vi "试验判定 - 副本.vi"(7 "Result":refnum<vi>, 10 "判定参数":T1, 11 "XY曲线":cluster{"X":dbl[], "Y":dbl[]}[](array[cluster])) -> (2 "判定项长度":i32, 3 "OK？":bool)   [LabVIEW 2020]
uses:
  Global_Variable/A131258.vi
  <userlib>/_MGI/1D Array/MGI Average/MGI Average (DBL[]).vi
panel:
  out "逆向平均值":dbl
  out "正向平均值":dbl
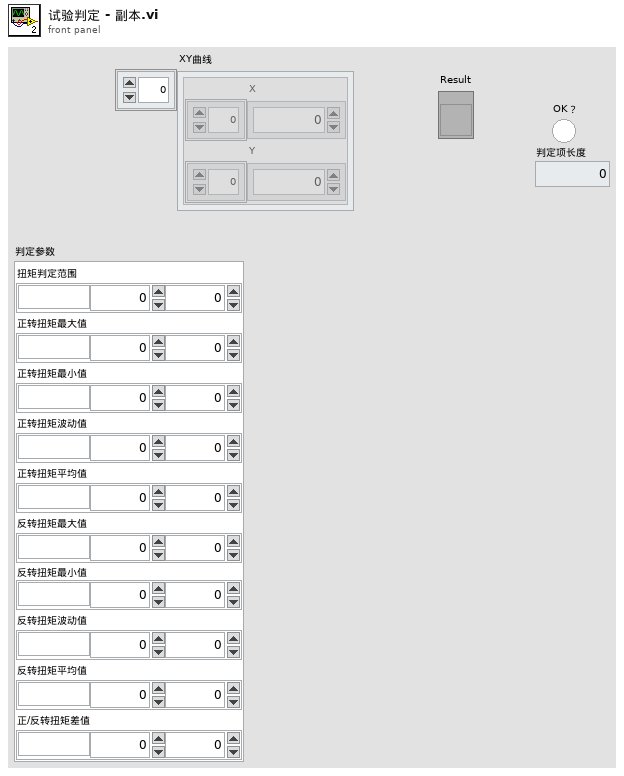
[diagram p1: front panel]
types:
  T1 = cluster{"扭矩判定范围":cluster{"单位":string, "下限":dbl, "上限":dbl}, "正转扭矩最大值":cluster{"单位":string, "下限":dbl, "上限":dbl}, "正转扭矩最小值":cluster{"单位":string, "下限":dbl, "上限":dbl}, "正转扭矩波动值":cluster{"单位":string, "下限":dbl, "上限":dbl}, "正转扭矩平均值":cluster{"单位":string, "下限":dbl, "上限":dbl}, "反转扭矩最大值":cluster{"单位":string, "下限":dbl, "上限":dbl}, "反转扭矩最小值":cluster{"单位":string, "下限":dbl, "上限":dbl}, "反转扭矩波动值":cluster{"单位":string, "下限":dbl, "上限":dbl}, "反转扭矩平均值":cluster{"单位":string, "下限":dbl, "上限":dbl}, "正/反转扭矩差值":cluster{"单位":string, "下限":dbl, "上限":dbl}}
  T2 = cluster{"左平均扭矩":cluster{"正转":dbl, "反转":dbl}, "左矩波动":cluster{"正转":dbl, "反转":dbl}, "左空载":cluster{"正转":dbl, "反转":dbl}, "右平均扭矩":cluster{"正转":dbl, "反转":dbl}, "右扭矩波动":cluster{"正转":dbl, "反转":dbl}, "右空载":cluster{"正转":dbl, "反转":dbl}, "扭矩对称":cluster{"左":dbl, "右":dbl}, "左零点漂移":cluster{"正":dbl, "反":dbl}, "右零点漂移":cluster{"正":dbl, "反":dbl}}
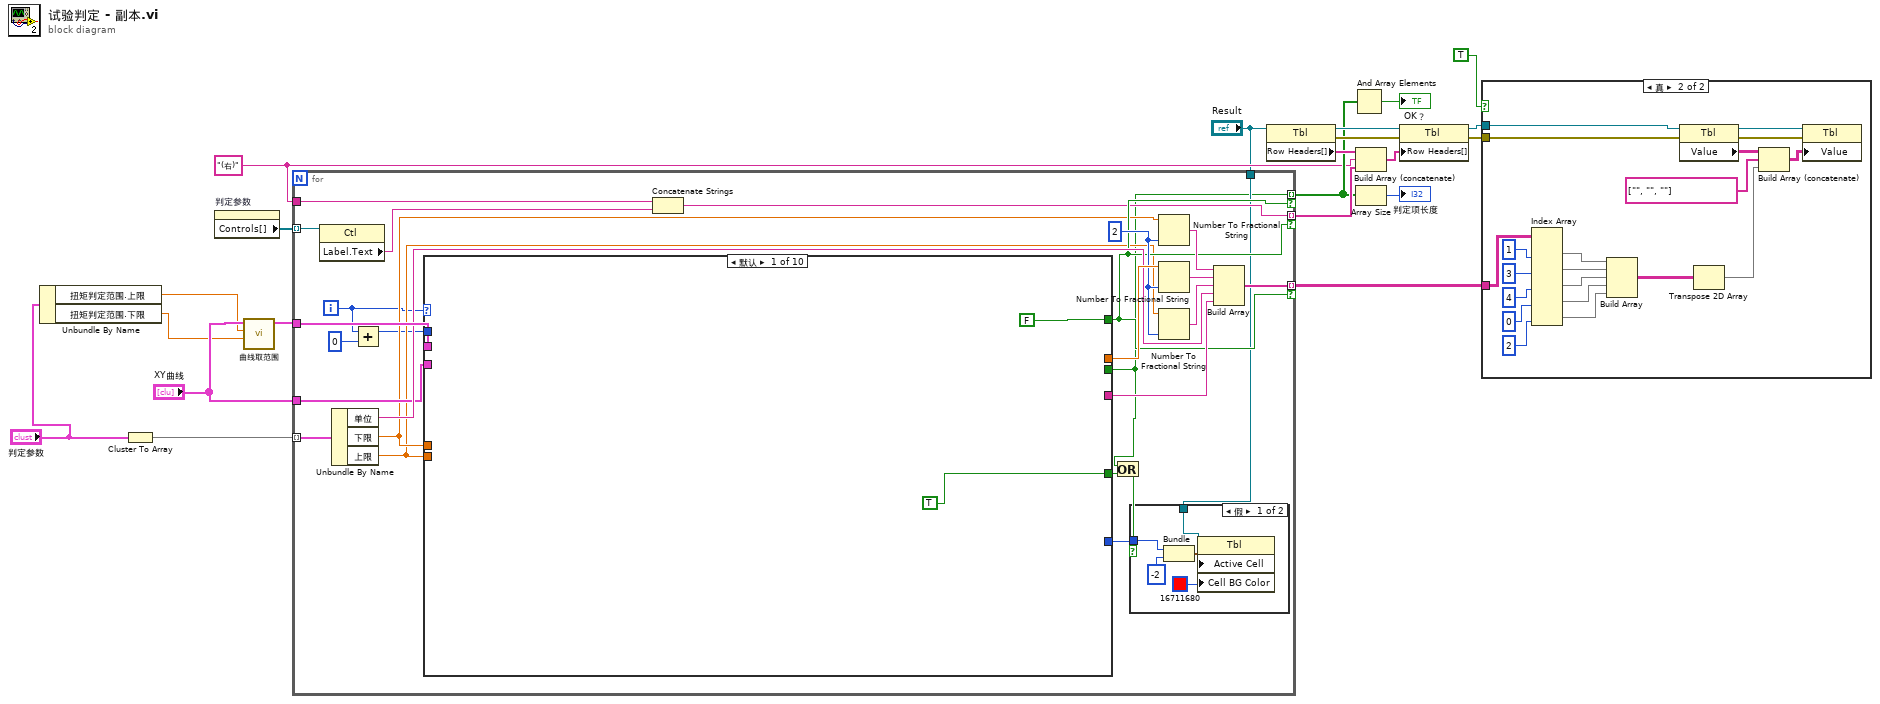
[diagram p0: block diagram]
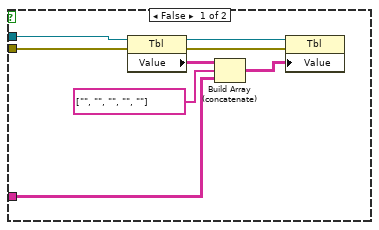
[diagram p2: hidden frame]
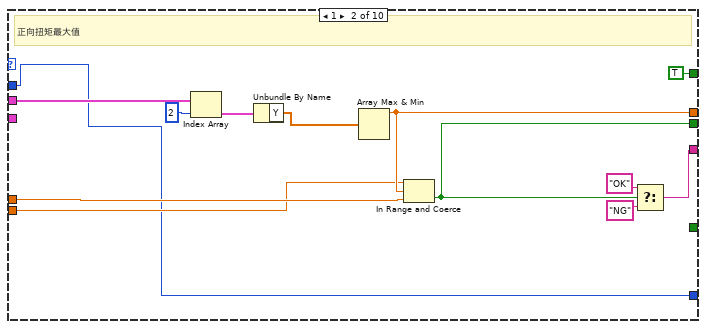
[diagram p4: hidden frame]
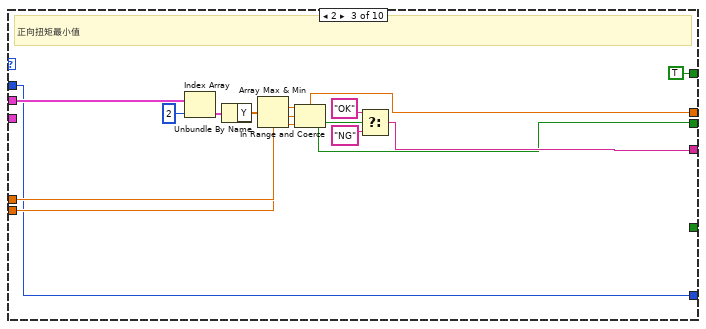
[diagram p5: hidden frame]
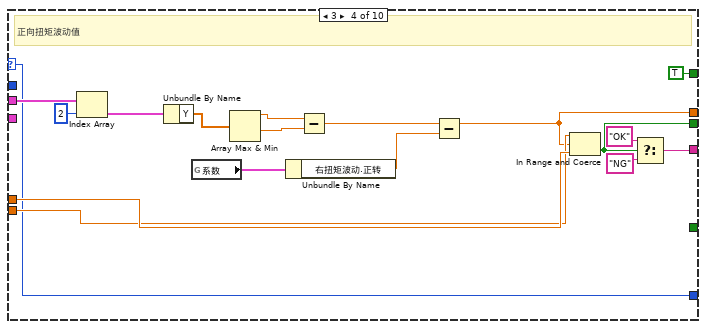
[diagram p6: hidden frame]
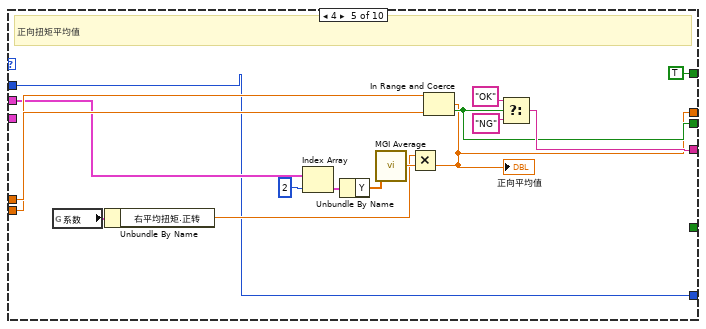
[diagram p7: hidden frame]
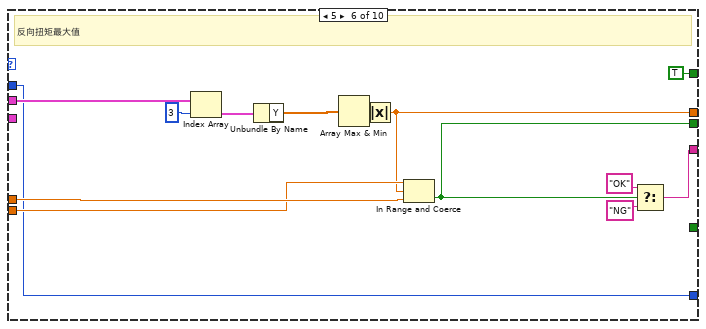
[diagram p8: hidden frame]
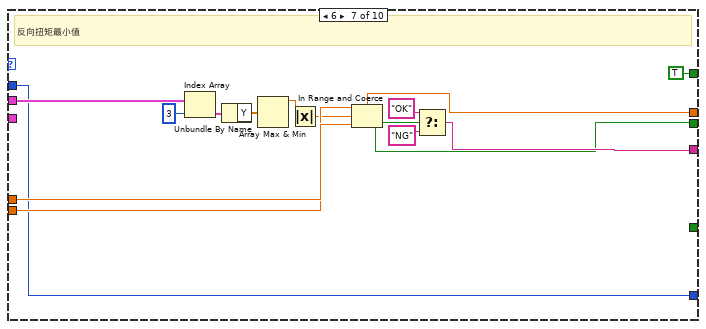
[diagram p9: hidden frame]
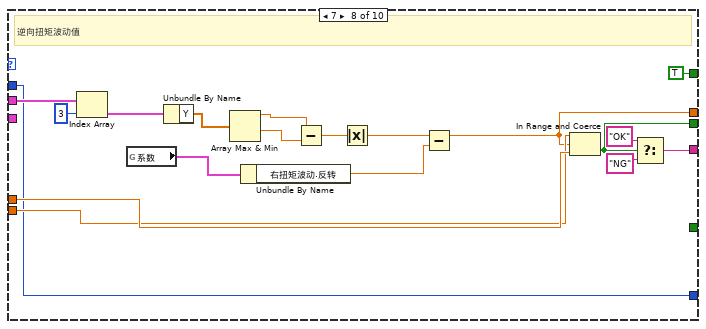
[diagram p10: hidden frame]
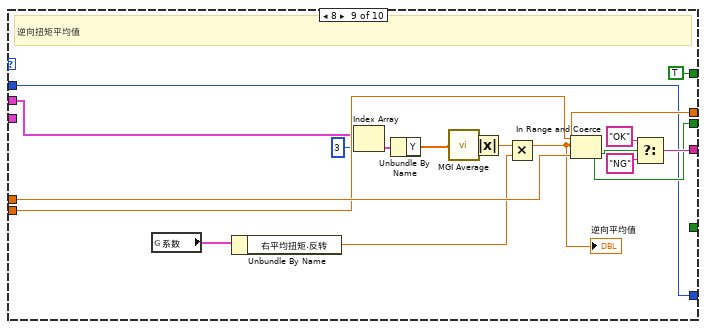
[diagram p11: hidden frame]
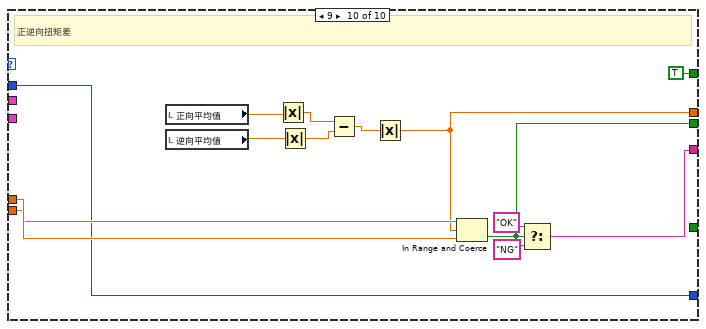
[diagram p12: hidden frame]
diagram:
  w7 = "(右)" ("Label.Text")
  n1 = Unbundle By Name("判定参数") -> ("扭矩判定范围.上限"=w2:dbl, "扭矩判定范围.下限"=w3:dbl)
  n2 = Cluster To Array(cluster="判定参数") -> (array=w21:cluster{"单位":string, "下限":dbl, "上限":dbl}[])
  n3 = property on="判定参数" class="Clust (严格)"() -> ("Controls[]"=w11:refnum<vi>[])  [unwired: 2 in, 2 out]
  n4 = call "曲线取范围.vi"("下限"=w3, "上限"=w2, "曲线In"="XY曲线") -> ("曲线Out"=w5:cluster{"X":dbl[], "Y":dbl[]}[])  [unwired: 8 in]
  n5 = for {
    tunnel: w21 -> [w47] mode=indexing
    tunnel: w11 -> [w46] mode=indexing
    tunnel: w5 -> [w44]
    tunnel: [w27] -> w9 mode=indexing if=w35
    tunnel: [w37] -> w12 mode=indexing if=w35
    tunnel: [w31] -> w14 mode=indexing if=w35
    tunnel: "XY曲线" -> [w34]
    tunnel: w7 -> [w30]
    tunnel: "Result" -> [w29]
    i -> [w23]
    w43 = i16 2 ("精度(6)")
    n6 = property class="Ctl"(reference=w46) -> ("Label.Text"=w36:string)  [unwired: 1 in, 2 out]
    n7 = Unbundle By Name(w47) -> ("单位"=w38:string, "下限"=w33:dbl, "上限"=w32:dbl)
    n8 = Add(x=w23, y=0) -> (x+y=w24:i32)
    n9 = case shown="默认" w23 {
      selector: w23 -> [_ _ _ w81 _ _ _ _ _ _]
      tunnel: [_ w64 w72 w83 w101 w117 w131 w145 w164 w181] -> w45
      tunnel: w44 -> [_ w67 w80 w92 w108 w128 w142 w155 w172 _]
      tunnel: [_ w61 w76 w96 w112 w123 w138 w159 w176 w182] -> w39
      tunnel: [_ w56 w69 w85 w103 w116 w130 w147 w166 w180] -> w27
      tunnel: w33 -> [_ w60 w75 w95 w111 w122 w137 w158 w175 w189]
      tunnel: w32 -> [_ w59 w74 w94 w110 w121 w136 w157 w174 w188]
      tunnel: [FALSE TRUE TRUE TRUE TRUE TRUE TRUE TRUE TRUE TRUE] -> w35
      tunnel: w34 -> [_ _ _ _ _ _ _ _ _ _]
      tunnel: [_ w55 w68 w81 w99 w115 w129 w143 w162 w179] -> w28
      tunnel: [TRUE _ _ _ _ _ _ _ _ _] -> w25
      tunnel: w24 -> [_ w55 w68 _ w99 w115 w129 w143 w162 w179]
      frame Default {
      }
      frame 1 {
        # "正向扭矩最大值"
        n10 = Index Array(array=w67, index=2 ("索引")) -> (element=w65:cluster{"X":dbl[], "Y":dbl[]})
        n11 = Unbundle By Name(w65) -> ("Y"=w57:dbl[])
        n12 = Array Max & Min(array=w57) -> (max value=w64:dbl)  [unwired: 3 out]
        n13 = In Range and Coerce(upper limit=w59, x=w64, lower limit=w60) -> (In Range?=w56:bool)  [unwired: 1 out]
        n14 = Select(t="OK", s=w56, f="NG") -> (s? t:f=w61:string)
      }
      frame 2 {
        # "正向扭矩最小值"
        n15 = Index Array(array=w80, index=2 ("索引")) -> (element=w79:cluster{"X":dbl[], "Y":dbl[]})
        n16 = Unbundle By Name(w79) -> ("Y"=w71:dbl[])
        n17 = Array Max & Min(array=w71) -> (min value=w72:dbl)  [unwired: 3 out]
        n18 = In Range and Coerce(upper limit=w74, x=w72, lower limit=w75) -> (In Range?=w69:bool)  [unwired: 1 out]
        n19 = Select(t="OK", s=w69, f="NG") -> (s? t:f=w76:string)
      }
      frame 3 {
        # "正向扭矩波动值"
        n20 = Index Array(array=w92, index=2 ("索引")) -> (element=w91:cluster{"X":dbl[], "Y":dbl[]})
        n21 = Unbundle By Name(w91) -> ("Y"=w89:dbl[])
        n22 = global read "A131258.vi" "系数"() -> (w84:T2)
        n23 = Array Max & Min(array=w89) -> (max value=w88:dbl, min value=w87:dbl)  [unwired: 2 out]
        n24 = Unbundle By Name(w84) -> ("右扭矩波动.正转"=w82:dbl)
        n25 = Subtract(x=w88, y=w87) -> (x-y=w86:dbl)
        n26 = Subtract(x=w86, y=w82) -> (x-y=w83:dbl)
        n27 = In Range and Coerce(upper limit=w94, x=w83, lower limit=w95) -> (In Range?=w85:bool)  [unwired: 1 out]
        n28 = Select(t="OK", s=w85, f="NG") -> (s? t:f=w96:string)
      }
      frame 4 {
        # "正向扭矩平均值"
        n29 = global read "A131258.vi" "系数"() -> (w102:T2)
        n30 = Unbundle By Name(w102) -> ("右平均扭矩.正转"=w100:dbl)
        n31 = Index Array(array=w108, index=2 ("索引")) -> (element=w107:cluster{"X":dbl[], "Y":dbl[]})
        n32 = Unbundle By Name(w107) -> ("Y"=w104:dbl[])
        n33 = call-poly <userlib>:"MGI Average.vi"("Double[]"=w104) -> ("Average"=w105:dbl)  [unwired: 1 in]
        n34 = Multiply(x=w100, y=w105) -> (x*y=w101:dbl)
        "正向平均值" <- w101
        n35 = In Range and Coerce(upper limit=w110, x=w101, lower limit=w111) -> (In Range?=w103:bool)  [unwired: 1 out]
        n36 = Select(t="OK", s=w103, f="NG") -> (s? t:f=w112:string)
      }
      frame 5 {
        # "反向扭矩最大值"
        n37 = Index Array(array=w128, index=3 ("索引")) -> (element=w126:cluster{"X":dbl[], "Y":dbl[]})
        n38 = Unbundle By Name(w126) -> ("Y"=w119:dbl[])
        n39 = Array Max & Min(array=w119) -> (min value=w118:dbl)  [unwired: 3 out]
        n40 = Absolute Value(x=w118) -> (abs(x)=w117:dbl)
        n41 = In Range and Coerce(upper limit=w121, x=w117, lower limit=w122) -> (In Range?=w116:bool)  [unwired: 1 out]
        n42 = Select(t="OK", s=w116, f="NG") -> (s? t:f=w123:string)
      }
      frame 6 {
        # "反向扭矩最小值"
        n43 = Index Array(array=w142, index=3 ("索引")) -> (element=w141:cluster{"X":dbl[], "Y":dbl[]})
        n44 = Unbundle By Name(w141) -> ("Y"=w134:dbl[])
        n45 = Array Max & Min(array=w134) -> (max value=w132:dbl)  [unwired: 3 out]
        n46 = Absolute Value(x=w132) -> (abs(x)=w131:dbl)
        n47 = In Range and Coerce(upper limit=w136, x=w131, lower limit=w137) -> (In Range?=w130:bool)  [unwired: 1 out]
        n48 = Select(t="OK", s=w130, f="NG") -> (s? t:f=w138:string)
      }
      frame 7 {
        # "逆向扭矩波动值"
        n49 = Index Array(array=w155, index=3 ("索引")) -> (element=w154:cluster{"X":dbl[], "Y":dbl[]})
        n50 = global read "A131258.vi" "系数"() -> (w146:T2)
        n51 = Unbundle By Name(w154) -> ("Y"=w152:dbl[])
        n52 = Array Max & Min(array=w152) -> (max value=w151:dbl, min value=w150:dbl)  [unwired: 2 out]
        n53 = Unbundle By Name(w146) -> ("右扭矩波动.反转"=w144:dbl)
        n54 = Subtract(x=w151, y=w150) -> (x-y=w149:dbl)
        n55 = Absolute Value(x=w149) -> (abs(x)=w148:dbl)
        n56 = Subtract(x=w148, y=w144) -> (x-y=w145:dbl)
        n57 = In Range and Coerce(upper limit=w157, x=w145, lower limit=w158) -> (In Range?=w147:bool)  [unwired: 1 out]
        n58 = Select(t="OK", s=w147, f="NG") -> (s? t:f=w159:string)
      }
      frame 8 {
        # "逆向扭矩平均值"
        n59 = global read "A131258.vi" "系数"() -> (w165:T2)
        n60 = Unbundle By Name(w165) -> ("右平均扭矩.反转"=w163:dbl)
        n61 = Index Array(array=w172, index=3 ("索引")) -> (element=w171:cluster{"X":dbl[], "Y":dbl[]})
        n62 = Unbundle By Name(w171) -> ("Y"=w170:dbl[])
        n63 = call-poly <userlib>:"MGI Average.vi"("Double[]"=w170) -> ("Average"=w168:dbl)  [unwired: 1 in]
        n64 = Absolute Value(x=w168) -> (abs(x)=w167:dbl)
        n65 = Multiply(x=w167, y=w163) -> (x*y=w164:dbl)
        "逆向平均值" <- w164
        n66 = In Range and Coerce(upper limit=w174, x=w164, lower limit=w175) -> (In Range?=w166:bool)  [unwired: 1 out]
        n67 = Select(t="OK", s=w166, f="NG") -> (s? t:f=w176:string)
      }
      frame 9 {
        # "正逆向扭矩差"
        n68 = local read "正向平均值"() -> (w187:dbl)
        n69 = local read "逆向平均值"() -> (w186:dbl)
        n70 = Absolute Value(x=w187) -> (abs(x)=w185:dbl)
        n71 = Absolute Value(x=w186) -> (abs(x)=w184:dbl)
        n72 = Subtract(x=w185, y=w184) -> (x-y=w183:dbl)
        n73 = Absolute Value(x=w183) -> (abs(x)=w181:dbl)
        n74 = In Range and Coerce(upper limit=w188, x=w181, lower limit=w189) -> (In Range?=w180:bool)  [unwired: 1 out]
        n75 = Select(t="OK", s=w180, f="NG") -> (s? t:f=w182:string)
      }
    }
    n76 = Concatenate Strings(w30, w36) -> (w31:string)
    n77 = Or(x=w27, y=w25) -> (x .or. y?=w26:bool)
    n78 = case shown="假" w26 {
      tunnel: w29 -> [w52 _]
      tunnel: w28 -> [w48 _]
      frame False {
        n79 = Bundle(w48, -2) -> (w50:cluster{i32, i32})  [unwired: 1 in]
        n80 = property class="Tbl"(reference=w52, "Active Cell"=w50, "Cell BG Color"=u32 16711680 ("活动单元格:单元格背景色")) -> ()  [unwired: 1 in, 2 out]
      }
      frame True {
      }
    }
    n81 = Number To Fractional String(number=w33, precision (6)=w43) -> (F-format string=w42:string)  [unwired: 2 in]
    n82 = Number To Fractional String(number=w45, precision (6)=w43) -> (F-format string=w41:string)  [unwired: 2 in]
    n83 = Number To Fractional String(number=w32, precision (6)=w43) -> (F-format string=w40:string)  [unwired: 2 in]
    n84 = Build Array(w42, w41, w40, w38, w39) -> (w37:string[])
  }
  n85 = property class="Tbl"(reference="Result") -> (reference out=w16:refnum<vi>, error out=w19:errorcluster, "Row Headers[]"=w13:string[])  [unwired: 1 in]
  n86 = And Array Elements(Boolean array=w9) -> (logical AND=→"OK？":bool)
  n87 = Build Array (concatenate)(w13, w7, w14) -> (w15:string[])
  n88 = Array Size(array=w9) -> (size(s)=→"判定项长度":i32)
  n89 = property class="Tbl"(reference=w16, error in=w19, "Row Headers[]"=w15) -> (reference out=w17:refnum<vi>, error out=w18:errorcluster)
  n90 = case shown="真" TRUE {
    tunnel: w18 -> [w198 w218]
    tunnel: w17 -> [w195 w215]
    tunnel: w12 -> [w194 w213]
    frame False {
      n91 = property class="Tbl"(reference=w195, error in=w198) -> (reference out=w196:refnum<vi>, error out=w197:errorcluster, "Value"=w199:string[][])
      n92 = Build Array (concatenate)(w199, string[] ["", "", "", "", ""], w194) -> (w200:string[][])
      n93 = property class="Tbl"(reference=w196, error in=w197, "Value"=w200) -> ()  [unwired: 2 out]
    }
    frame True {
      n94 = Index Array(array=w213, index (col) #1=1 ("禁用的索引 (列)"), index (col) #2=3 ("索引 (列)"), index (col) #3=4 ("索引 (列)"), index (col) #4=0 ("索引 (列)"), index (col) #5=2 ("索引 (列)")) -> (element #1=w209:string[], element #2=w208:string[], element #3=w207:string[], element #4=w202:string[], element #5=w201:string[])  [unwired: 5 in]
      n95 = Build Array(w209, w208, w207, w202, w201) -> (w206:string[][])
      n96 = property class="Tbl"(reference=w215, error in=w218) -> (reference out=w216:refnum<vi>, error out=w217:errorcluster, "Value"=w219:string[][])
      n97 = Transpose 2D Array(2D array=w206) -> (transposed array=w205:string[][])
      n98 = Build Array (concatenate)(w219, string[] ["", "", ""], w205) -> (w220:string[][])
      n99 = property class="Tbl"(reference=w216, error in=w217, "Value"=w220) -> ()  [unwired: 2 out]
    }
  }
